vi "wait.vi"(0 "HGF_DSCEvent":refnum<class "HGF_DSCEvent.lvclass">, 3 "msTimeout (-1)":i32=-1, 5 "error in (no error)":errorcluster, 9 "ignore previous (F)":bool) -> (14 "dup HGF_DSCEvent":refnum<class "HGF_DSCEvent.lvclass">, 16 "Object":refnum<class>, 17 "timed out":bool, 19 "error out":errorcluster)   [LabVIEW 2012, in "HGF_DSC.lvlib" / "HGF_DSCEvent.lvclass"]
doc: "Use this VI to wait on events.\n\n<b>Hint:</b> This is a shared reentrant VI."
uses:
  HGF_DSCEvent.lvclass
  HGF_DSCEvent.lvclass/HGF_DSCEvent.ctl
  HGF_BaseClasses/HGF_NetworkVisitor/HGF_NetworkVisitor.lvclass
  HGF_BaseClasses/HGF_Event/HGF_Event.lvclass
  HGF_BaseClasses/HGF_Timing/HGF_Timing.lvclass
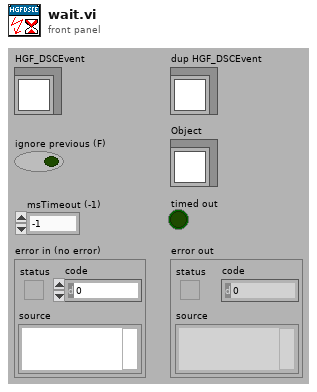
[diagram p1: front panel]
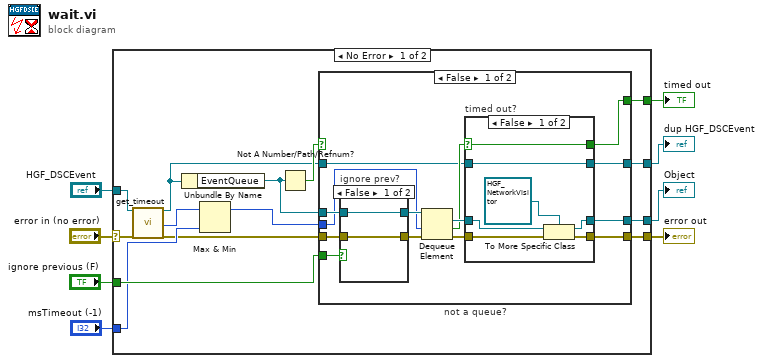
[diagram p0: block diagram]
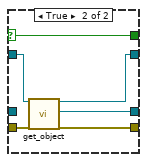
[diagram p2: hidden frame]
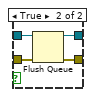
[diagram p3: hidden frame]
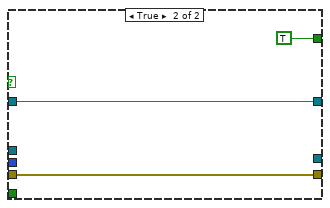
[diagram p4: hidden frame]
diagram:
  n1 = case shown="No Error" "error in (no error)" {
    selector: "error in (no error)" -> [w14 w60]
    tunnel: "HGF_DSCEvent" -> [w18 w59]
    tunnel: [w9 w59] -> w7
    tunnel: "msTimeout (-1)" -> [w16 _]
    tunnel: "ignore previous (F)" -> [w20 _]
    tunnel: [w22 _] -> w3
    tunnel: [w21 w60] -> w2
    tunnel: [w19 _] -> w1
    frame No Error {
      n2 = call "get_timeout.vi"("HGF_Event.lvclass in"=w18, "error in (no error)"=w14) -> ("HGF_Event.lvclass out"=w10:refnum<class "HGF_DSCEvent.lvclass">, "timeout"=w17:i32, "error out"=w13:errorcluster)  [unwired: 15 out]
      n3 = Unbundle By Name(w10) -> ("EventQueue"=w12:refnum<queue>)
      n4 = Max & Min(x=w17, y=w16) -> (max(x,y)=w15:i32)  [unwired: 1 out]
      n5 = Not A Number/Path/Refnum?(number/path/refnum=w12) -> (NaN/Path/Refnum?=w11:bool)
      n6 = case "not a queue?" shown="False" w11 {
        tunnel: [w36 _] -> w22
        tunnel: [w35 w57] -> w21
        tunnel: w12 -> [w33 _]
        tunnel: w20 -> [w31 _]
        tunnel: [w28 TRUE] -> w19
        tunnel: w15 -> [w26 _]
        tunnel: w13 -> [w25 w57]
        tunnel: w10 -> [w24 w58]
        tunnel: [w23 w58] -> w9
        frame False {
          n7 = case "ignore prev?" shown="False" w31 {
            tunnel: w33 -> [w51 w55]
            tunnel: [w51 w54] -> w32
            tunnel: w25 -> [w50 w53]
            tunnel: [w50 w52] -> w30
            frame False {
            }
            frame True {
              n8 = Flush Queue(queue=w55, error in (no error)=w53) -> (queue out=w54:refnum<queue>, error out=w52:errorcluster)  [unwired: 1 out]
            }
          }
          n9 = Dequeue Element(queue=w32, timeout in ms (-1)=w26, error in (no error)=w30) -> (element=w34:refnum<class "HGF_NetworkVisitor.lvclass">, timed out?=w29:bool, error out=w27:errorcluster)  [unwired: 1 out]
          n10 = case "timed out?" shown="False" w29 {
            selector: w29 -> [w40 w49]
            tunnel: [w43 w46] -> w36
            tunnel: [w42 w44] -> w35
            tunnel: w34 -> [w41 _]
            tunnel: [w40 w49] -> w28
            tunnel: w27 -> [w39 w45]
            tunnel: w24 -> [w38 w48]
            tunnel: [w38 w47] -> w23
            frame False {
              n11 = To More Specific Class(target class=refnum<class "HGF_NetworkVisitor.lvclass"> refnum ("HGF_BaseClasses.lvlib:HGF_NetworkVisitor.lvclass"), reference=w41, error in=w39) -> (specific class reference=w43:refnum<class "HGF_NetworkVisitor.lvclass">, error out=w42:errorcluster)
            }
            frame True {
              n12 = call "get_object.vi"("HGF_Timing.lvclass"=w48, "error in (no error)"=w45) -> ("dup HGF_Timing"=w47:refnum<class "HGF_DSCEvent.lvclass">, "object"=w46:refnum<class>, "error out"=w44:errorcluster)  [unwired: 15 out]
            }
          }
        }
        frame True {
        }
      }
    }
    frame Error {
    }
  }
  "error out" <- w2
  "dup HGF_DSCEvent" <- w7
  "timed out" <- w1
  "Object" <- w3
